vi "TSLIN_Receive.vi"(10 "路径输入":path) -> (3 "ALINData":T1)   [LabVIEW 2019]
uses:
  Typedef/TLibLIN.ctl
panel:
  out "tsapp_transmit_header_and_receive_msg":i32
  out "路径输出":path
  in  "ATimeoutMs":i32
  in  "ADLC":u8
  in  "AIdentifier":u8 format="%x"
  in  "AChn":i32
  in  "TLIBLIN":T1
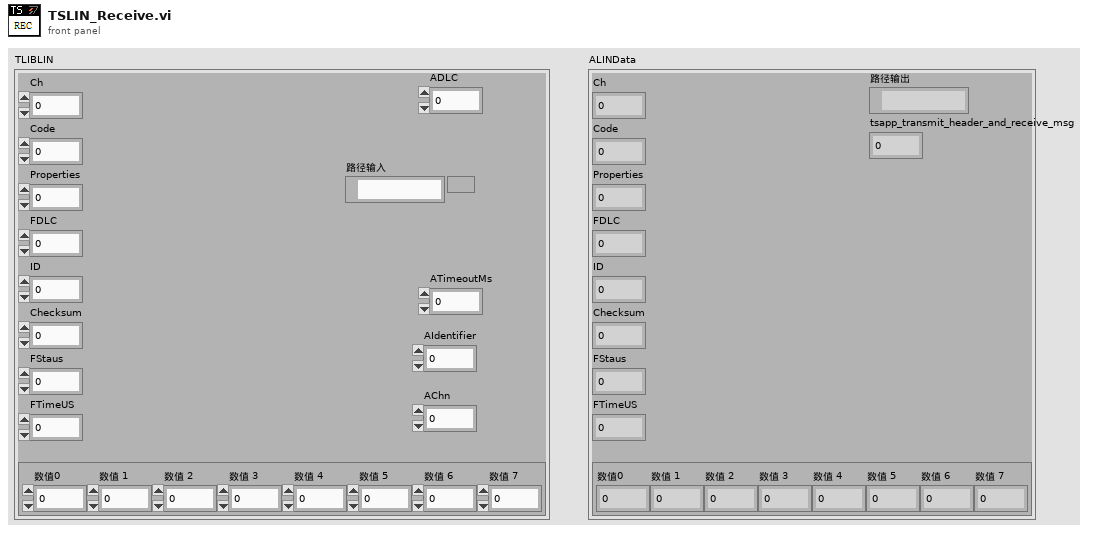
[diagram p1: front panel]
types:
  T1 = typedef "TLibLIN.ctl" = cluster{"Ch":u8, "Code":u8, "Properties":u8, "FDLC":u8, "ID":u8, "Checksum":u8, "FStaus":u8, "FTimeUS":u64, "FDatas":cluster{"数值0":u8, "数值 1":u8, "数值 2":u8, "数值 3":u8, "数值 4":u8, "数值 5":u8, "数值 6":u8, "数值 7":u8}}
  T2 = cluster{"数值0":u8, "数值 1":u8, "数值 2":u8, "数值 3":u8, "数值 4":u8, "数值 5":u8, "数值 6":u8, "数值 7":u8}
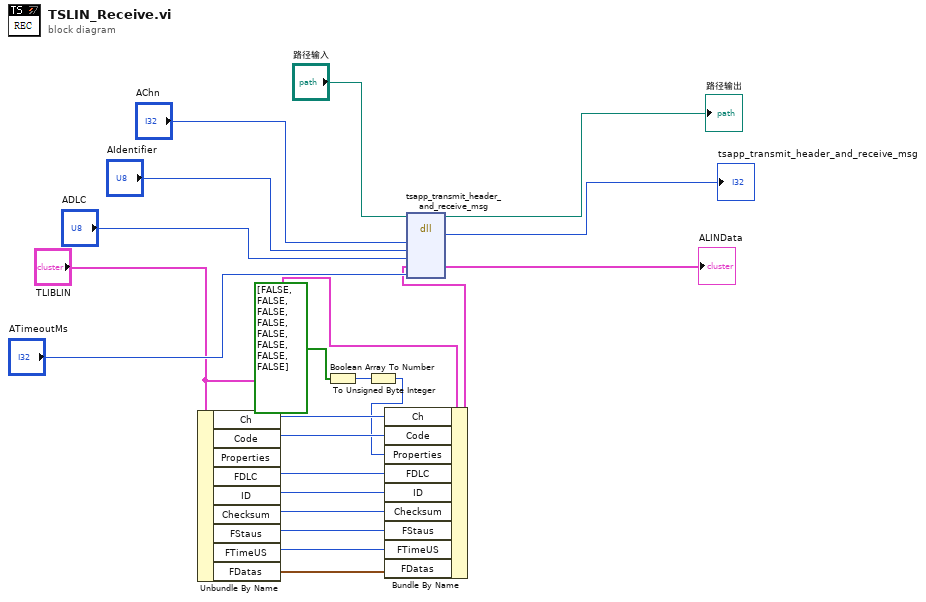
[diagram p0: block diagram]
diagram:
  n1 = Unbundle By Name("TLIBLIN") -> ("Ch"=w13:u8, "Code"=w12:u8, "FDLC"=w11:u8, "ID"=w10:u8, "Checksum"=w9:u8, "FStaus"=w8:u8, "FTimeUS"=w7:u64, "FDatas"=w1:T2)  [unwired: 1 out]
  n2 = Boolean Array To Number(Boolean array=bool[] [FALSE, FALSE, FALSE, FALSE, FALSE, FALSE, FALSE, FALSE]) -> (number=w6:u32)
  n3 = To Unsigned Byte Integer(number=w6) -> (unsigned 8bit integer=w4:u8)
  n4 = Bundle By Name(cluster="TLIBLIN", "Ch"=w13, "Code"=w12, "Properties"=w4, "FDLC"=w11, "ID"=w10, "Checksum"=w9, "FStaus"=w8, "FTimeUS"=w7, "FDatas"=w1) -> (w3:T1)
  n5 = dll-call lib="PTH2@abs EDemo同星TSCAN_V1.4_20220301ConfigTSMaster.dll" fn="tsapp_transmit_header_and_receive_msg"(path in="路径输入", "AChn"="AChn", "AIdentifier"="AIdentifier", "ADLC"="ADLC", "ALINData"=w3, "ATimeoutMs"="ATimeoutMs") -> (path out=→"路径输出":path, "tsapp_transmit_header_and_receive_msg"=→"tsapp_transmit_header_and_receive_msg":i32, "ALINData"=→"ALINData":T1)  [unwired: 6 in, 1 out]
